vi "FromExample.vi"() -> ()   [LabVIEW 2018, in "Pid.lvlib"]
uses:
  Pid.lvlib
  <vilib>/addons/control/pid/NI_PID_autopid.lvlib
panel:
  out "Modbus Error":errorcluster
  out "Output":dbl(knob) scale=0.0..260.0
  in  "Instructions":string="Overview: This example demonstrates how to use a PID Autotuning for systems with large delay, by using the Internal Model Control algorithm for first-order model with transport delay (deadtime).\nInstructions:\n1. Run the VI and wait until the process variable (PV) reaches near setpoint (SP).\n2.  On the PID Autotuning Design section, select the  type of controller, step amplitude for the 'open loop step response'. Then, press Identify and tune to start the process.\n3.  When the tuned PID gains do not change anymore or the indicator tuning completed? flashes, the identification is done and you can accept new gains by pressing Accept gain. That will transfer the new gain to PID Gains.\n4. Click Identify and tune again to go back to the automatic control. You can try different options and repeat this process. Time constant factor specifies a divider to apply to the identified time constant to obtain the desired time constant response. Time constant factor to a value greater than 1 makes the desired time constant used in the design faster (more aggressive). Time constant factor to a value less than 1 makes the response slower (more conservative).\nStep amplitude specifies the amplitude of the step applied to the open loop identification.  \n5. Click Stop to stop the VI.\n"
  in  "Stop":bool
  out "SP and PV":cluster{"initial PV":dbl, "SP1:":dbl}(graph)={"initial PV"=50.98160323470328, "SP1:"=50.98039215686275}
  in  "Sampling Time dt (s)":dbl=0.1 min=0.001 step=0.01 format="%#.3p"
  in  "PID Gains":T1={"proportional gain (Kc)"=1.0198114826651394, "integral time (Ti, min)"=0.06332676917403887, "derivative time (Td, min)"=0.0} {"derivative time (Td, min)" format="%#.6g"; "integral time (Ti, min)" format="%#.6g"; "proportional gain (Kc)" format="%#.6g"}
  in  "SP1:":dbl(slide)=37.254901960784316 min=0.0 max=0.0 scale=0.0..100.0
  out "PV1:":dbl(slide)=42.840793682454986 scale=0.0..100.0
  in  "MV1:":dbl(slide)=15.081495361740814 scale=-100.0..100.0
  in  "Identify and tune":bool
  out "MV":dbl(graph)=20.39115328927357
  in  "autotuning parameters":T2={"type of controller"=1, "time constant factor"=2.0, "step amplitude"=1.0} {"time constant factor" scale=0.0001..1000.0; "step amplitude" format="%.2f"; "type of controller" items=["P", "PI", "PID"]}
  in  "Reinitialize":bool
  in  "Automatic":bool=TRUE
  in  "initial plant parameters":T3={"process gain"=2.515490777679412, "time constant (s)"=2.529236380296785, "delay time (s)"=2.5407395402910935} {"delay time (s)" format="%.3f"; "time constant (s)" format="%.3f"; "process gain" format="%.3f"}
  out "tuning completed?":bool
  in  "Alpha":dbl(slide) scale=0.0..1.0
  in  "Accept gain":bool
  out "tuned PID gains":T1={"proportional gain (Kc)"=15.221889907608013, "integral time (Ti, min)"=0.002027201803862475, "derivative time (Td, min)"=0.0002815558060920104} {"derivative time (Td, min)" format="%#.6g"; "integral time (Ti, min)" format="%#.6g"; "proportional gain (Kc)" format="%#.6g"}
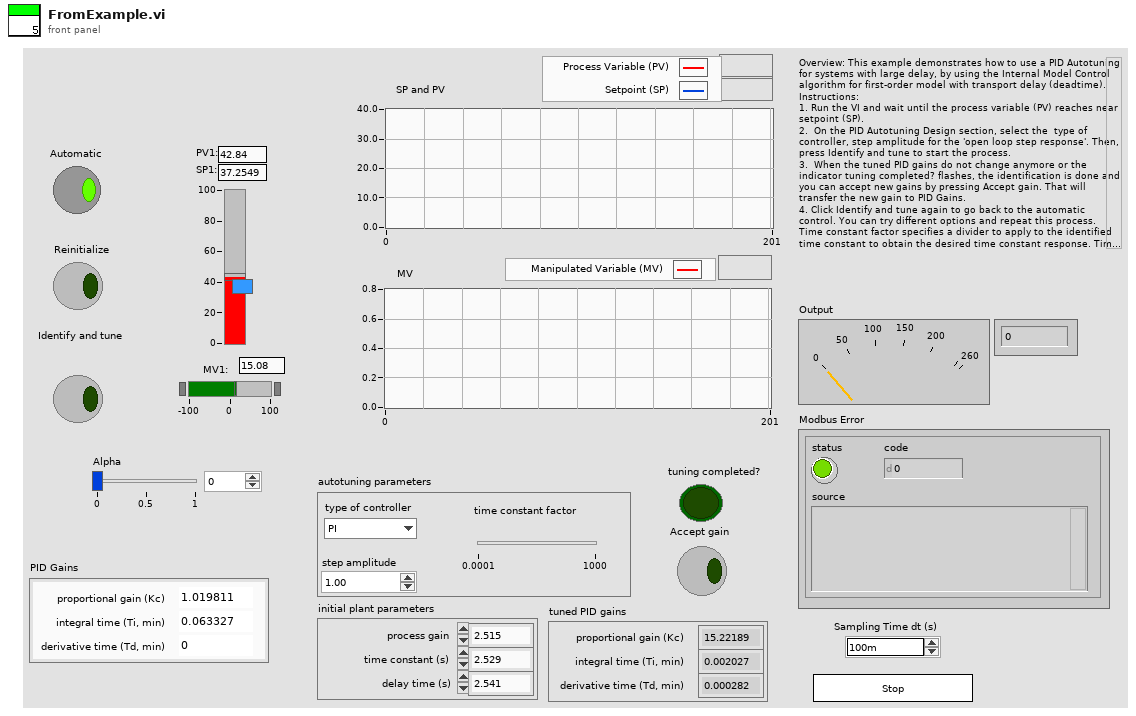
[diagram p1: front panel]
types:
  T1 = cluster{"proportional gain (Kc)":dbl, "integral time (Ti, min)":dbl, "derivative time (Td, min)":dbl}
  T2 = cluster{"type of controller":u16, "time constant factor":dbl, "step amplitude":dbl}
  T3 = cluster{"process gain":dbl, "time constant (s)":dbl, "delay time (s)":dbl}
  T4 = cluster{"static gain":dbl, "lag (s)":dbl, "deadtime (s)":dbl, "load":dbl, "deadband":dbl, "sensor noise":dbl, "initial PV":dbl, "plant noise":dbl}
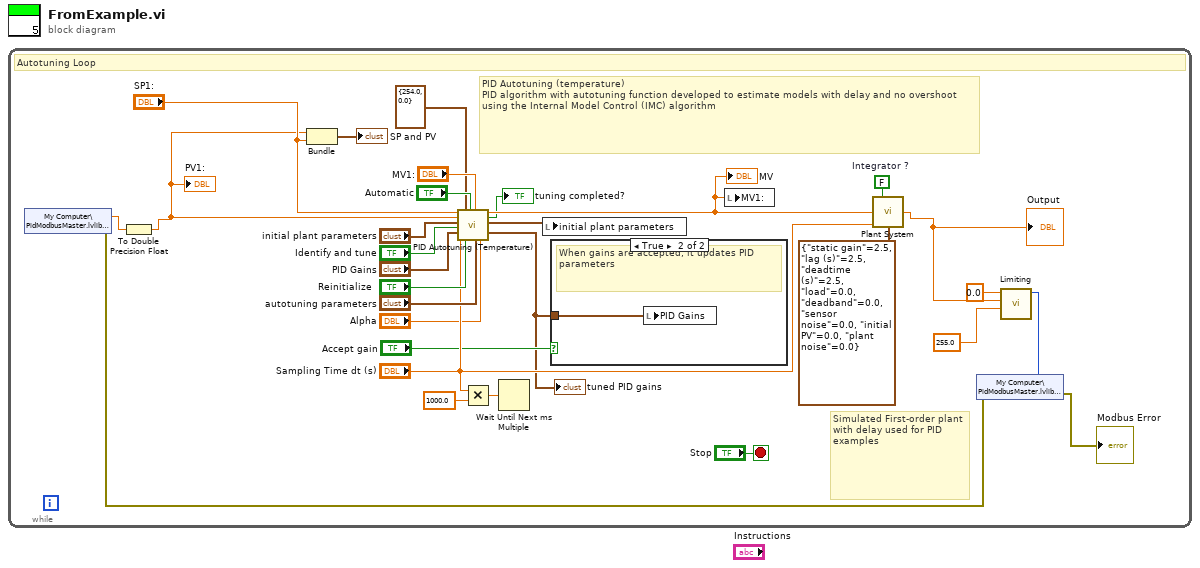
[diagram p0: block diagram]
diagram:
  n1 = while {
    stop <- "Stop" stop-if-true
    w19 = FALSE  # Integrator ?
    # "PID Autotuning (temperature)\nPID algorithm with autotuning function developed to estimate models with delay and no overshoot using the Internal Model Control (IMC) algorithm"
    # "Simulated First-order plant with delay used for PID examples"
    # "Autotuning Loop"
    n2 = shared-variable "My Computer\\PidModbusMaster.lvlib\\F300002"() -> (w9:sgl, error out=w1:errorcluster)  [unwired: 1 in]
    n3 = To Double Precision Float(number=w9) -> (double precision float=w8:dbl)
    "PV1:" <- w8
    n4 = Bundle(w8, "SP1:"="SP1:") -> (→"SP and PV":cluster{dbl, "SP1:":dbl})  [unwired: 1 in]
    n5 = call <vilib>:"PID Autotuning (Temperature).vi"("desired temperature"="SP1:", "measured temperature"=w8, "plant parameters in"="initial plant parameters", "autotune? (F)"="Identify and tune", "PID gains in"="PID Gains", "dt (s)"="Sampling Time dt (s)", "output range"=cluster{"output high":dbl, "output low":dbl} {"output high"=254.0, "output low"=0.0}, "reinitialize? (F)"="Reinitialize", "auto? (T)"="Automatic", "manual control"="MV1:", "autotuning parameters"="autotuning parameters", "alpha"="Alpha") -> ("output"=w23:dbl, "tuning completed?"=→"tuning completed?":bool, "plant parameters out"=w17:T3, "PID gains out"=w12:T1)  [unwired: 4 in]
    "MV" <- w23
    "tuned PID gains" <- w12
    n6 = Multiply(x="Sampling Time dt (s)", y=1000.0 ("Numeric")) -> (x*y=w11:dbl)
    n7 = Wait Until Next ms Multiple(millisecond multiple=w11) -> ()  [unwired: 1 out]
    n8 = local write "initial plant parameters"(w17) -> ()
    n9 = case shown="True" "Accept gain" {
      tunnel: w12 -> [_ w31]
      frame False {
        # "otherwise, do nothing"
      }
      frame True {
        # "When gains are accepted, it updates PID parameters"
        n10 = local write "PID Gains"(w31) -> ()
      }
    }
    n11 = local write "MV1:"(w23) -> ()
    n12 = call "Plant System.vi"("Integrator ?"=w19, "Plant Input"=w23, "dt (s)"="Sampling Time dt (s)", "process parameters"=T4 {"static gain"=2.5, "lag (s)"=2.5, "deadtime (s)"=2.5, "load"=0.0, "deadband"=0.0, "sensor noise"=0.0, "initial PV"=0.0, "plant noise"=0.0} ("plant parameters")) -> ("Plant Output"=w7:dbl)  [unwired: 11 in]
    "Output" <- w7
    n13 = call "Limiting.vi"("Maximum"=255.0, "Value"=w7, "Minimum"=0.0) -> ("Output"=w3:i16)  [unwired: 8 in]
    n14 = shared-variable "My Computer\\PidModbusMaster.lvlib\\S400001"(w3, error in=w1) -> (error out=→"Modbus Error":errorcluster)
  }
